vi "camera-write_trigger-source-acquisition-start.vi"(6 "error in (no error)":errorcluster, 8 "Option":T1(ring), 9 "IMAQ Session In":refnum<k11>) -> (0 "error out":errorcluster, 1 "Data":string, 2 "Address":string, 3 "IMAQ Session Out":refnum<k11>)   [LabVIEW 2012]
panel:
  out "Loop Iteration":i32
  out "ACK/NAK":string
  out "String to Write":string
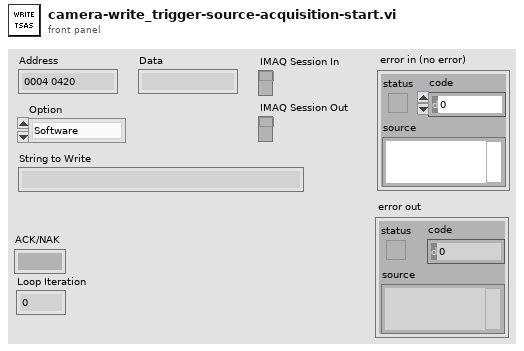
[diagram p1: front panel]
types:
  T1 = enum16{"Software", "Line1", "Line2", "CC1", "CC2", "CC3", "CC4"}
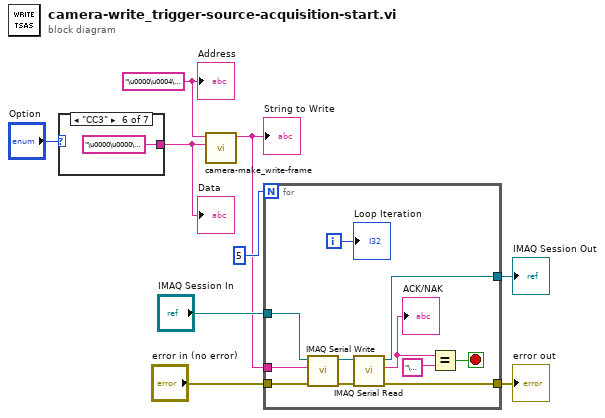
[diagram p0: block diagram]
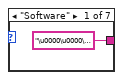
[diagram p2: hidden frame]
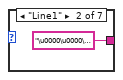
[diagram p3: hidden frame]
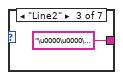
[diagram p4: hidden frame]
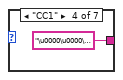
[diagram p5: hidden frame]
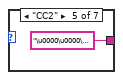
[diagram p6: hidden frame]
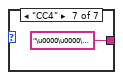
[diagram p7: hidden frame]
diagram:
  w2 = "\u0000\u0004\u0001@" ("Address")
  n1 = case shown="\"CC3\"" "Option" {
    tunnel: ["\u0000\u0000\u0000\u0000" ("Address") "\u0000\u0000\u0000\u0001" ("Address") "\u0000\u0000\u0000\u0002" ("Address") "\u0000\u0000\u0000\t" ("Address") "\u0000\u0000\u0000\n" ("Address") "\u0000\u0000\u0000\u000b" ("Address") "\u0000\u0000\u0000\f" ("Address")] -> w1
    frame "Software" {
    }
    frame "Line1" {
    }
    frame "Line2" {
    }
    frame "CC1" {
    }
    frame "CC2" {
    }
    frame "CC3" {
    }
    frame "CC4" {
    }
  }
  "Data" <- w1
  n2 = call "camera-make_write-frame.vi"("Data"=w1, "Address"=w2) -> ("Serial String"=w7:string)  [unwired: 9 in]
  "String to Write" <- w7
  n3 = for {
    N: 5 -> [_]
    tunnel: "IMAQ Session In" -> [w27]
    tunnel: w7 -> [w26]
    tunnel: [w25] -> w6
    tunnel: "error in (no error)" -> [w24]
    tunnel: [w22] -> w4
    i -> [w18]
    stop <- w21 stop-if-true
    n4 = call <vilib>:"IMAQ Serial Write.vi"("error in (no error)"=w24, "String to write"=w26, "IMAQ Session In"=w27) -> ("error out"=w23:errorcluster, "IMAQ Session Out"=w17:refnum<k11>)  [unwired: 5 in]
    n5 = call <vilib>:"IMAQ Serial Read.vi"("error in (no error)"=w23, "IMAQ Session In"=w17) -> ("error out"=w22:errorcluster, "String Read"=w20:string, "IMAQ Session Out"=w25:refnum<k11>)  [unwired: 4 in, 1 out]
    "ACK/NAK" <- w20
    n6 = Equal?(x=w20, y="\u0006") -> (x = y?=w21:bool)
    "Loop Iteration" <- w18
  }
  "IMAQ Session Out" <- w6
  "error out" <- w4
  "Address" <- w2
